vi "certaintyGraph.vi"(8 "Detected":bool, 9 "Y":u16, 10 "X":i16, 11 "Array":i16[][](array[numeric])) -> (3 "Array 2":i16[][](array[numeric]))   [LabVIEW 2012]
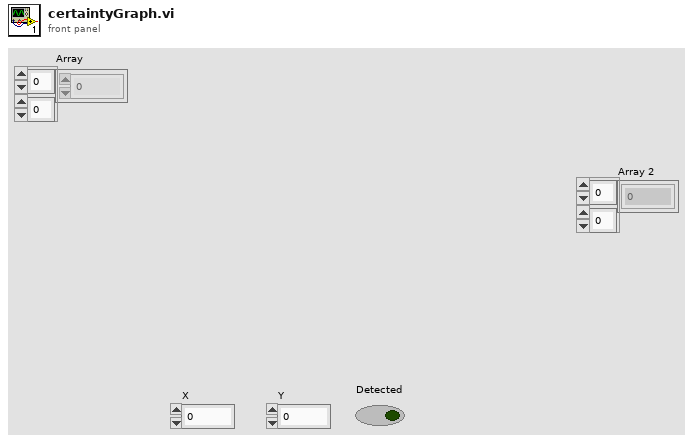
[diagram p1: front panel]
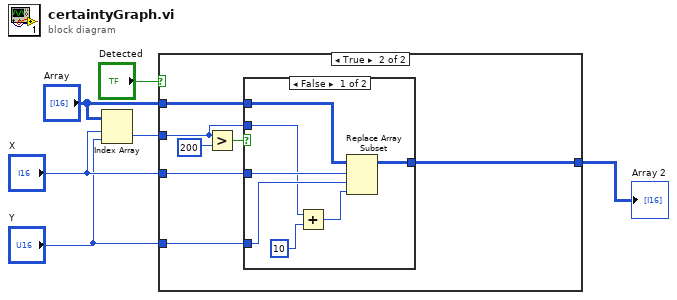
[diagram p0: block diagram]
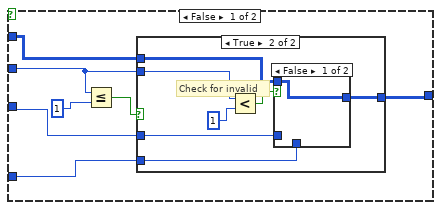
[diagram p2: hidden frame]
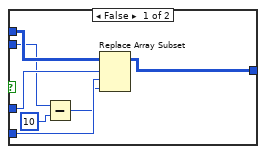
[diagram p3: hidden frame]
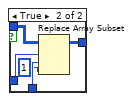
[diagram p4: hidden frame]
diagram:
  n1 = Index Array(array="Array", index (row)="X", index (col)="Y") -> (element=w5:i16)
  n2 = case shown="True" "Detected" {
    tunnel: w5 -> [w11 w35]
    tunnel: "Array" -> [w10 w40]
    tunnel: "X" -> [w9 w39]
    tunnel: "Y" -> [w8 w38]
    tunnel: [w7 w34] -> w1
    frame False {
      n3 = Less Or Equal?(x=w11, y=1) -> (x <= y?=w12:bool)
      n4 = case shown="True" w12 {
        tunnel: w11 -> [w15 w27]
        tunnel: w10 -> [w20 w24]
        tunnel: w9 -> [w18 w23]
        tunnel: w8 -> [w17 w22]
        tunnel: [w19 w21] -> w7
        frame False {
          n5 = Subtract(x=w15, y=10) -> (x-y=w14:i32)
          n6 = Replace Array Subset(array=w20, new element=w14, index (row)=w18, index (col)=w17) -> (w19:i16[][])
        }
        frame True {
          # "Check for invalid"
          n7 = Less?(x=w27, y=1) -> (x < y?=w25:bool)
          n8 = case shown="False" w25 {
            tunnel: w24 -> [w28 w33]
            tunnel: w23 -> [_ w32]
            tunnel: w22 -> [_ w31]
            tunnel: [w28 w29] -> w21
            frame False {
            }
            frame True {
              n9 = Replace Array Subset(array=w33, new element=1, index (row)=w32, index (col)=w31) -> (w29:i16[][])
            }
          }
        }
      }
    }
    frame True {
      n10 = Greater?(x=w35, y=200) -> (0:w36:bool)
      n11 = case shown="False" w36 {
        tunnel: w40 -> [w43 w48]
        tunnel: w39 -> [w47 _]
        tunnel: w38 -> [w46 _]
        tunnel: w35 -> [w45 _]
        tunnel: [w41 w48] -> w34
        frame False {
          n12 = Add(x=w45, y=10) -> (x+y=w44:i32)
          n13 = Replace Array Subset(array=w43, new element=w44, index (row)=w47, index (col)=w46) -> (w41:i16[][])
        }
        frame True {
          # "Certainty cant go higher"
        }
      }
    }
  }
  "Array 2" <- w1
